vi "Find Frame Time.vi"(1 "Status":T1) -> (0 "Frame Time (ms)":i32)   [LabVIEW 2020]
uses:
  Status Cluster STYP.ctl
  Snake/Snake.lvclass
  INIFile/INIScoreFile.lvclass
  Drawing Settings STYP.ctl
  Food/Food.lvclass
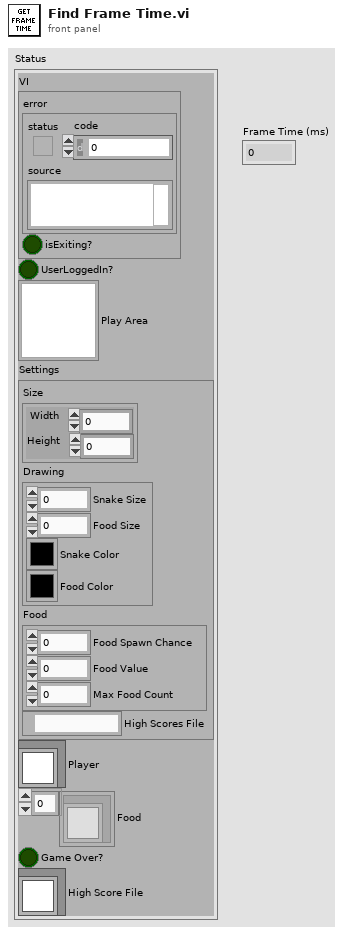
[diagram p1: front panel]
types:
  T1 = typedef "Status Cluster STYP.ctl" = cluster{"VI":cluster{"error":errorcluster, "isExiting?":bool}, "UserLoggedIn?":bool, "Play Area":picture, "Settings":cluster{"Size":cluster{"Width":u32, "Height":u32}, "Drawing":T2, "Food":cluster{"Food Spawn Chance":dbl, "Food Value":u32, "Max Food Count":i32}, "High Scores File":path}, "Player":refnum<class "Snake.lvclass">, "Food":refnum<class "Food.lvclass">[], "Game Over?":bool, "High Score File":refnum<class "INIScoreFile.lvclass">}
  T2 = typedef "Drawing Settings STYP.ctl" = cluster{"Snake Size":u32, "Food Size":u32, "Snake Color":u32, "Food Color":u32}
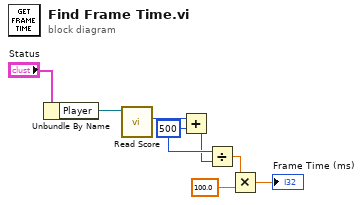
[diagram p0: block diagram]
diagram:
  w5 = u32 500 ("y")
  n1 = Unbundle By Name("Status") -> ("Player"=w7:refnum<class "Snake.lvclass">)
  n2 = call-dynamic "Read Score.vi"("Snake in"=w7) -> ("Score"=w6:u32)  [unwired: 8 in, 2 out]
  n3 = Add(x=w6, y=w5) -> (x+y=w4:u32)
  n4 = Divide(x=w5, y=w4) -> (x/y=w3:dbl)
  n5 = Multiply(x=w3, y=100.0) -> (x*y=→"Frame Time (ms)":dbl)
